vi "processor.vi"(10 "application request":T1={"request id"=0, "role"=enum."none", "standard input"="", "data"="", "dictionary"=variant(cluster{"key":string, "value":string}[] []), "close after response"=FALSE}, 11 "connection":refnum<k5>) -> ()   [LabVIEW 2013]
uses:
  application request.ctl
  begin request role.ctl
  record types.ctl
  end request body.ctl
  end request protocol status.ctl
  record header.ctl
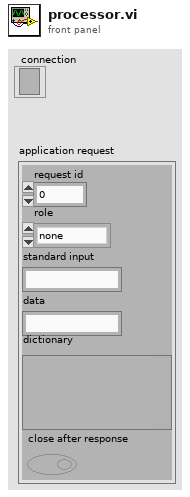
[diagram p1: front panel]
types:
  T1 = typedef "application request.ctl" = cluster{"request id":u16, "role":T2, "standard input":string, "data":string, "dictionary":variant, "close after response":bool}
  T2 = typedef "begin request role.ctl" = enum16{"none", "Responder", "Authorizer", "Filter"}
  T3 = typedef "record header.ctl" = cluster{"version":u8, "type":T4, "request id":u16, "content length":u16, "padding length":u8, "reserved":u8}
  T4 = typedef "record types.ctl" = enum8{"Error", "Begin Request", "Abort Request", "End Request", "Parameters", "Standard Input", "Standard Output", "Standard Error", "Data", "Get Values", "Get Values Result", "Unknown Type"}
  T5 = typedef "end request protocol status.ctl" = enum8{"complete", "cant mpx connection", "overloaded", "unknown role"}
  T6 = typedef "end request body.ctl" = cluster{"application status":u32, "protocol status":T5, "reserved 1":u8, "reserved 2":u8, "reserved 3":u8}
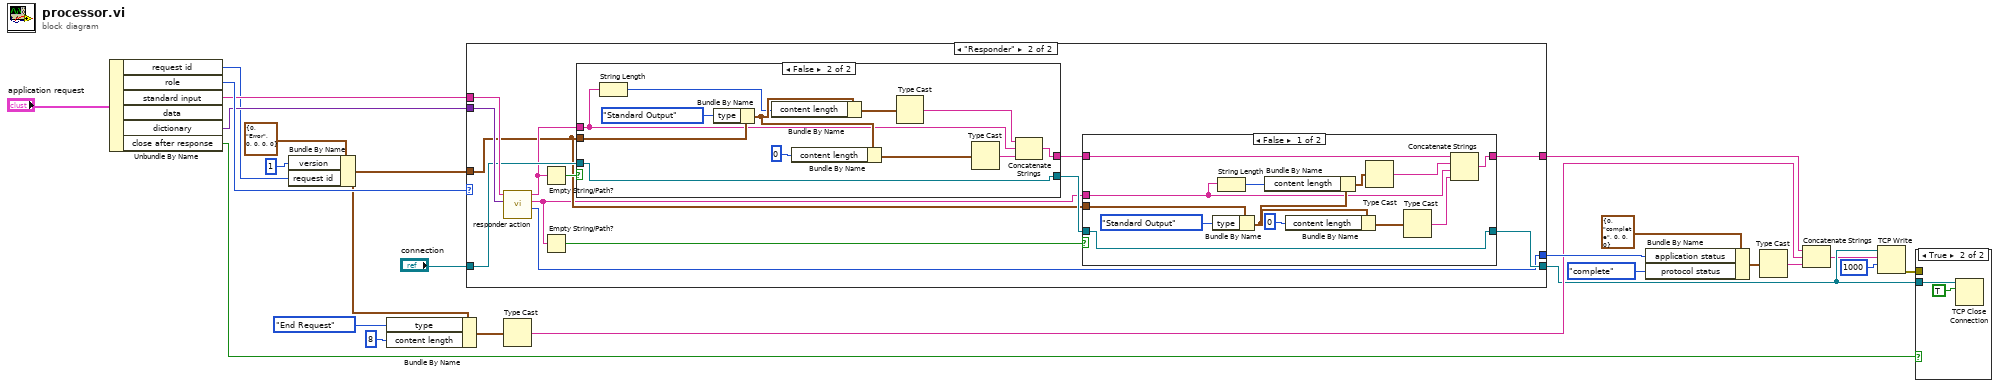
[diagram p0: block diagram]
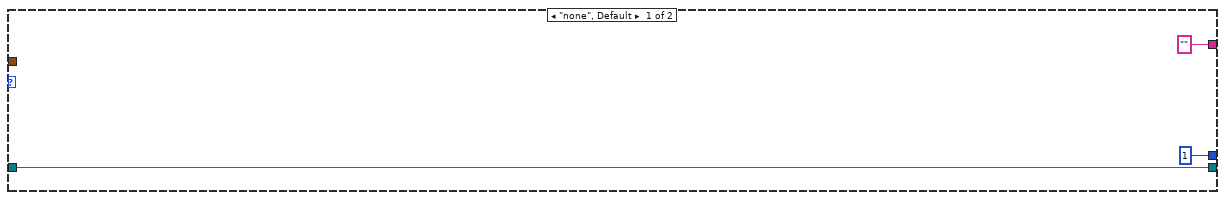
[diagram p3: hidden frame]
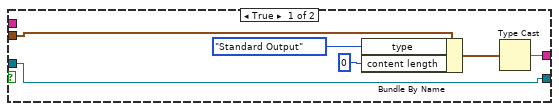
[diagram p5: hidden frame]
diagram:
  n1 = Unbundle By Name("application request") -> ("request id"=w12:u16, "role"=w23:T2, "standard input"=w20:string, "dictionary"=w19:variant, "close after response"=w21:bool)  [unwired: 1 out]
  n2 = Bundle By Name(cluster=T3 {"version"=0, "type"=enum."Error", "request id"=0, "content length"=0, "padding length"=0, "reserved"=0} ("header"), "version"=u8 1, "request id"=w12) -> (w11:T3)
  n3 = Bundle By Name(cluster=w11, "type"=record_types."End Request", "content length"=u16 8) -> (w6:T3)
  n4 = case shown="\"Responder\"" w23 {
    tunnel: "connection" -> [w27 w37]
    tunnel: [w27 w35] -> w3
    tunnel: w20 -> [_ w40]
    tunnel: w19 -> [_ w39]
    tunnel: w11 -> [_ w32]
    tunnel: [u32 1 ("code") w30] -> w9
    tunnel: ["" w28] -> w5
    frame "none", Default {
    }
    frame "Responder" {
      n5 = call "responder action.vi"("dictionary"=w39, "standard input"=w40) -> ("code"=w30:u32, "standard error"=w31:string, "standard out"=w33:string)  [unwired: 7 in]
      n6 = Empty String/Path?(string/path=w33) -> (empty?=w38:bool)
      n7 = Empty String/Path?(string/path=w31) -> (empty?=w36:bool)
      n8 = case shown="False" w38 {
        tunnel: w32 -> [w60 w72]
        tunnel: w37 -> [w59 w71]
        tunnel: [w59 w71] -> w34
        tunnel: w33 -> [_ w63]
        tunnel: [w56 w62] -> w29
        frame True {
          n9 = Bundle By Name(cluster=w60, "type"=record_types."Standard Output", "content length"=u16 0) -> (w57:T3)
          n10 = Type Cast(x=w57) -> (*(type *) &x=w56:string)  [unwired: 1 in]
        }
        frame False {
          n11 = String Length(string=w63) -> (length=w68:i32)
          n12 = Bundle By Name(cluster=w72, "type"=record_types."Standard Output") -> (w70:T3)
          n13 = Bundle By Name(cluster=w70, "content length"=w68) -> (w64:T3)
          n14 = Bundle By Name(cluster=w70, "content length"=u16 0) -> (w65:T3)
          n15 = Type Cast(x=w64) -> (*(type *) &x=w67:string)  [unwired: 1 in]
          n16 = Type Cast(x=w65) -> (*(type *) &x=w66:string)  [unwired: 1 in]
          n17 = Concatenate Strings(w67, w63, w66) -> (w62:string)
        }
      }
      n18 = case shown="False" w36 {
        tunnel: [w48 w55] -> w35
        tunnel: w34 -> [w48 w55]
        tunnel: w32 -> [w49 _]
        tunnel: w31 -> [w41 _]
        tunnel: w29 -> [w45 w54]
        tunnel: [w44 w54] -> w28
        frame False {
          n19 = Bundle By Name(cluster=w49, "type"=record_types."Standard Output") -> (w51:T3)
          n20 = String Length(string=w41) -> (length=w53:i32)
          n21 = Bundle By Name(cluster=w51, "content length"=w53) -> (w42:T3)
          n22 = Bundle By Name(cluster=w51, "content length"=u16 0) -> (w43:T3)
          n23 = Type Cast(x=w42) -> (*(type *) &x=w46:string)  [unwired: 1 in]
          n24 = Type Cast(x=w43) -> (*(type *) &x=w47:string)  [unwired: 1 in]
          n25 = Concatenate Strings(w45, w46, w41, w47) -> (w44:string)
        }
        frame True {
        }
      }
    }
  }
  n26 = Type Cast(x=w6) -> (*(type *) &x=w8:string)  [unwired: 1 in]
  n27 = Bundle By Name(cluster=T6 {"application status"=0, "protocol status"=enum."complete", "reserved 1"=0, "reserved 2"=0, "reserved 3"=0} ("record header"), "application status"=w9, "protocol status"=end_request_protocol_status."complete") -> (w16:T6)
  n28 = Type Cast(x=w16) -> (*(type *) &x=w7:string)  [unwired: 1 in]
  n29 = Concatenate Strings(w5, w8, w7) -> (w2:string)
  n30 = TCP Write(connection ID=w3, data in=w2, 9:1000 ("timeout ms (25000)")) -> (error out=w4:errorcluster)  [unwired: 1 in, 2 out]
  n31 = case shown="True" w21 {
    tunnel: w3 -> [_ w74]
    tunnel: w4 -> [_ _]
    frame False {
    }
    frame True {
      n32 = TCP Close Connection(connection ID=w74, abort (F)=TRUE) -> ()  [unwired: 1 in, 2 out]
    }
  }
